vi "Launch Plot.vi"(8 "error in (no error)":errorcluster, 9 "Plot type":T1, 10 "File Path Control":path, 11 "Measure Controller in":refnum<class "Process Controller.lvclass">) -> (0 "error out":errorcluster, 2 "Nested Actor's Enqueuer":refnum<class "Message Enqueuer.lvclass">, 3 "Measure Controller out":refnum<class "Process Controller.lvclass">)   [LabVIEW 2016, in "Process Controller.lvclass"]
uses:
  Process Controller.lvclass
  Plots/Plot types.ctl
  <vilib>/ActorFramework/Message Enqueuer/Message Enqueuer.lvclass
  Plots/XY WFRM Plot/XY WFRM Plot.lvclass
  D:/github/Measure_core/Plots/Plot/Plot.lvclass
  Plots/XY WFRM Plot/XY WFRM Plot.lvclass/XY WFRM Plot.ctl
  Plots/XY Plot/XY Plot.lvclass
  Process Controller.lvclass/Process Controller.ctl
  Plots/Plot Messages/Add file Msg/Add file Msg.lvclass/Add file Msg.ctl
  <vilib>/ActorFramework/Message Enqueuer/Message Enqueuer.lvclass/Message Enqueuer.ctl
  Plots/XY WFRM Plot/Write Plot type.vi
  <vilib>/ActorFramework/Message Enqueuer/Enqueue.vi
  Plots/Plot/Plot.lvclass
  D:/github/Measure_core/Measure Object/Measure Object.lvclass
  Plots/Plot Messages/Add file Msg/Add file Msg.lvclass
  D:/Program Files/National Instruments/LabVIEW 2016/vi.lib/ActorFramework/Message/Message.lvclass
  Measure Object Messages/Open Front Panel Msg/Open Front Panel Msg.lvclass
  <vilib>/ActorFramework/Message Priority Queue/Priority Enqueue.vi
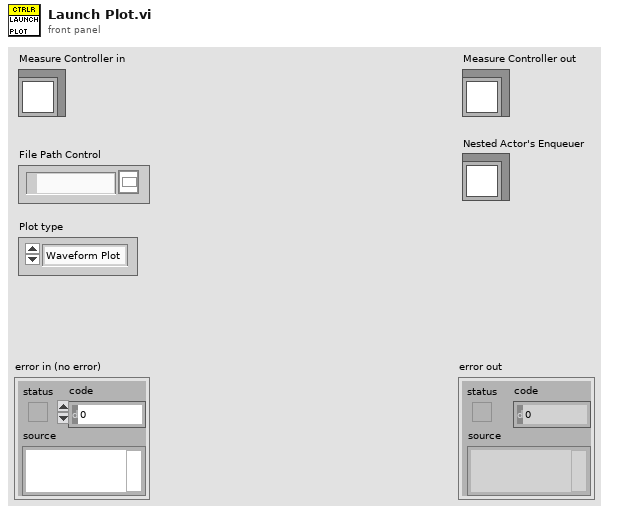
[diagram p1: front panel]
types:
  T1 = typedef "Plot types.ctl" = enum16{"Waveform Plot", "XY Plot", "Full XY"}
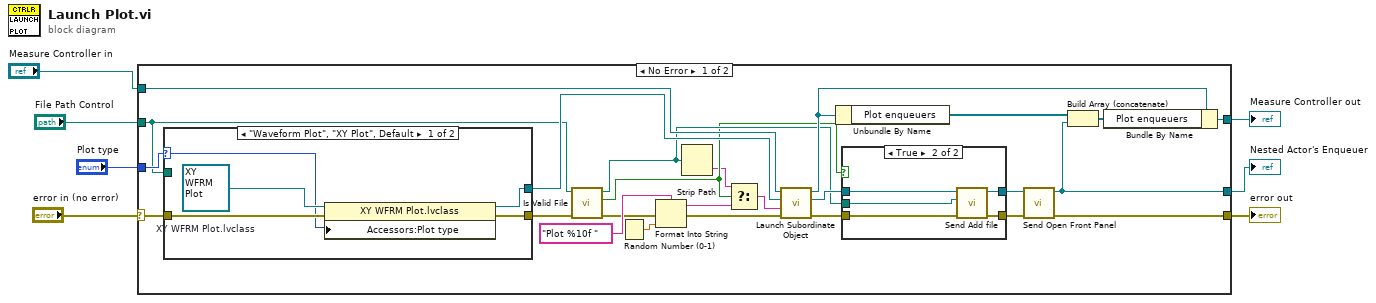
[diagram p0: block diagram]
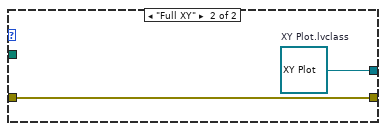
[diagram p3: hidden frame]
diagram:
  n1 = case shown="No Error" "error in (no error)" {
    selector: "error in (no error)" -> [w30 w48]
    tunnel: [w31 w48] -> w6
    tunnel: [w23 w47] -> w4
    tunnel: "Measure Controller in" -> [w32 w47]
    tunnel: "File Path Control" -> [w19 _]
    tunnel: "Plot type" -> [w26 _]
    tunnel: [w20 _] -> w1
    frame No Error {
      n2 = case shown="\"Waveform Plot\", \"XY Plot\", Default" w26 {
        selector: w26 -> [w40 _]
        tunnel: [w42 w46] -> w29
        tunnel: w19 -> [_ _]
        tunnel: [w41 w45] -> w18
        tunnel: w30 -> [w43 w45]
        frame "Waveform Plot", "XY Plot", Default {
          w44 = refnum<class "XY WFRM Plot.lvclass"> refnum  # XY WFRM Plot.lvclass
          n3 = property class="XY WFRM Plot.lvclass"(reference=w44, error in=w43, "Accessors:Plot type"=w40) -> (reference out=w42:refnum<class "XY WFRM Plot.lvclass">, error out=w41:errorcluster)
        }
        frame "Full XY" {
          w46 = refnum<class "XY Plot.lvclass"> refnum  # XY Plot.lvclass
        }
      }
      n4 = call "Is Valid File.vi"("Error In"=w18, "File"=w19) -> ("Error Out"=w8:errorcluster, "Valid file"=w15:bool, "File out"=w16:path)  [unwired: 7 in]
      n5 = Random Number (0-1)() -> (number: 0 to 1=w13:dbl)
      n6 = Format Into String(format string="Plot %10f ", error in=w8, w13) -> (resulting string=w11:string, error out=w9:errorcluster)  [unwired: 1 in]
      n7 = Strip Path(path=w16) -> (name=w14:string)  [unwired: 1 out]
      n8 = Select(t=w14, s=w15, f=w11) -> (s? t:f=w10:string)
      n9 = call-dynamic "Launch Subordinate Object.vi"("error in (no error)"=w9, "Name"=w10, "Subordinate Object"=w29, "Measure Object in"=w32) -> ("error out"=w17:errorcluster, "Nested Actor's Enqueuer"=w28:refnum<class "Message Enqueuer.lvclass">, "Measure Object out"=w24:refnum<class "Process Controller.lvclass">)  [unwired: 5 in]
      n10 = Unbundle By Name(w24) -> ("Plot enqueuers"=w22:refnum<class "Message Enqueuer.lvclass">[])
      n11 = case shown="True" w15 {
        tunnel: w28 -> [w34 w39]
        tunnel: [w34 w38] -> w27
        tunnel: [w33 w37] -> w25
        tunnel: w17 -> [w33 w36]
        tunnel: w16 -> [_ w35]
        frame False {
        }
        frame True {
          n12 = call "Send Add file.vi"("error in (no error)"=w36, "File Path Control"=w35, "Message Enqueuer"=w39) -> ("error out"=w37:errorcluster, "Message Enqueuer out"=w38:refnum<class "Message Enqueuer.lvclass">)  [unwired: 7 in]
        }
      }
      n13 = call "Send Open Front Panel.vi"("error in (no error)"=w25, "Message Enqueuer"=w27) -> ("error out"=w31:errorcluster, "Message Enqueuer out"=w20:refnum<class "Message Enqueuer.lvclass">)  [unwired: 8 in]
      n14 = Build Array (concatenate)(w22, w20) -> (w21:refnum<class "Message Enqueuer.lvclass">[])
      n15 = Bundle By Name(cluster=w24, "Plot enqueuers"=w21) -> (w23:refnum<class "Process Controller.lvclass">)
    }
    frame Error {
    }
  }
  "error out" <- w6
  "Measure Controller out" <- w4
  "Nested Actor's Enqueuer" <- w1
